vi "test_F9P.vi"() -> ()   [LabVIEW 2019] (continued)
085,36,09,44,196,30,11,78,037,33,2*7B\r\n$GAGSV,3,2,09,12,32,115,24,18,55,284,37,19,17,042,30,25,01,241,,2*76\r\n$GAGSV,3,3,09,36,35,314,26,2*4E\r\n$GBGSV,4,1,13,04,35,133,,05,09,257,,06,27,182,,07,09,201,,1*7B\r\n$GBGSV,4,2,13,08,65,355,39,09,07,194,,10,16,222,23,11,37,142,25,1*73\r\n$GBGSV,4,3,13,13,50,315,40,14,76,037,42,28,59,310,38,33,73,239,30,1*71\r\n$GBGSV,4,4,13,34,13,142,,1*46\r\n$GBGSV,4,1,13,04,35,133,,05,09,257,,06,27,182,,07,09,201,,3*79\r\n$GBGSV,4,2,13,08,65,355,38,09,07,194,,10,16,222,26,11,37,142,35,3*74\r\n$GBGSV,4,3,13,13,50,315,42,14,76,037,38,28,59,310,,33,73,239,,3*74\r\n$GBGSV,4,4,13,34,13,142,,3*44\r\n$GNGLL,3723.61677,N,12656.96875,E,064301.00,A,A*70\r\n$GNRMC,064302.00,A,3723.61678,N,12656.96879,E,0.043,,250720,,,A,V*16\r\n$GNVTG,,T,,M,0.043,N,0.079,K,A*34\r\n$GNGGA,064302.00,3723.61678,N,12656.96879,E,1,12,0.63,44.0,M,18.5,M,,*7F\r\n$GNGSA,A,3,17,19,06,05,02,12,09,,,,,,1.10,0.63,0.91,1*09\r\n$GNGSA,A,3,85,70,71,72,,,,,,,,,1.10,0.63,0.91,2*06\r\n$GNGSA,A,3,36,19,11,04,09,12,,,,,,,1.10,0.63,0.91,3*0D\r\n$GNGSA,A,3,28,14,13,11,33,08,10,,,,,,1.10,0.63,0.91,4*0D\r\n$GPGSV,4,1,13,02,65,334,45,04,08,037,36,05,48,261,35,06,58,076,45,1*6B\r\n$GPGSV,4,2,13,07,06,105,,09,38,057,49,12,18,263,22,13,08,191,21,1*65\r\n$GPGSV,4,3,13,17,19,158,26,19,37,161,28,25,11,294,,29,07,323,21,1*62\r\n$GPGSV,4,4,13,30,01,134,,1*52\r\n$GPGSV,4,1,13,02,65,334,,04,08,037,21,05,48,261,32,06,58,076,24,6*6B\r\n$GPGSV,4,2,13,07,06,105,10,09,38,057,40,12,18,263,12,13,08,191,,6*6A\r\n$GPGSV,4,3,13,17,19,158,17,19,37,161,,25,11,294,,29,07,323,,6*6E\r\n$GPGSV,4,4,13,30,01,134,,6*55\r\n$GLGSV,2,1,06,70,55,030,38,71,68,223,32,72,17,216,36,84,09,133,12,1*7C\r\n$GLGSV,2,2,06,85,63,111,36,86,51,337,,1*7F\r\n$GLGSV,2,1,06,70,55,030,,71,68,223,18,72,17,216,22,84,09,133,12,3*78\r\n$GLGSV,2,2,06,85,63,111,28,86,51,337,19,3*7A\r\n$GAGSV,3,1,09,02,04,287,09,04,68,085,42,09,44,196,31,11,78,037,39,7*7F\r\n$GAGSV,3,2,09,12,32,115,28,18,55,284,35,19,17,042,34,25,01,241,,7*79\r\n$GAGSV,3,3,09,36,35,314,33,7*4F\r\n$GAGSV,3,1,09,02,04,287,,04,68,085,36,09,44,196,26,11,78,037,33,2*7C\r\n$GAGSV,3,2,09,12,32,115,24,18,55,284,38,19,17,042,30,25,01,241,,2*79\r\n$GAGSV,3,3,09,36,35,314,26,2*4E\r\n$GBGSV,4,1,13,04,35,133,,05,09,257,,06,27,182,,07,09,201,,1*7B\r\n$GBGSV,4,2,13,08,65,355,40,09,07,194,,10,16,222,22,11,37,142,22,1*7B\r\n$GBGSV,4,3,13,13,50,315,40,14,76,037,42,28,59,310,38,33,73,239,32,1*73\r\n$GBGSV,4,4,13,34,13,142,,1*46\r\n$GBGSV,4,1,13,04,35,133,,05,09,257,,06,27,182,,07,09,201,,3*79\r\n$GBGSV,4,2,13,08,65,355,38,09,07,194,,10,16,222,26,11,37,142,34,3*75\r\n$GBGSV,4,3,13,13,50,315,41,14,76,037,37,28,59,310,,33,73,239,,3*78\r\n$GBGSV,4,4,13,34,13,142,,3*44\r\n$GNGLL,3723.61678,N,12656.96879,E,064302.00,A,A*70\r\n$GNRMC,064303.00,A,3723.61679,N,12656.96883,E,0.052,,250720,,,A,V*13\r\n$GNVTG,,T,,M,0.052,N,0.096,K,A*35\r\n$GNGGA,064303.00,3723.61679,N,12656.96883,E,1,12,0.63,44.1,M,18.5,M,,*7B\r\n$GNGSA,A,3,17,19,06,05,02,12,09,,,,,,1.10,0.63,0.91,1*09\r\n$GNGSA,A,3,85,70,71,72,,,,,,,,,1.10,0.63,0.91,2*06\r\n$GNGSA,A,3,36,19,11,04,09,12,,,,,,,1.10,0.63,0.91,3*0D\r\n$GNGSA,A,3,28,14,13,11,33,08,10,,,,,,1.10,0.63,0.91,4*0D\r\n$GPGSV,4,1,13,02,65,334,44,04,08,037,33,05,48,261,31,06,58,076,44,1*6A\r\n$GPGSV,4,2,13,07,06,105,,09,38,057,49,12,18,263,22,13,08,191,21,1*65\r\n$GPGSV,4,3,13,17,19,158,26,19,37,161,28,25,11,294,,29,07,323,20,1*63\r\n$GPGSV,4,4,13,30,01,134,,1*52\r\n$GPGSV,4,1,13,02,65,334,,04,08,037,22,05,48,261,32,06,58,076,26,6*6A\r\n$GPGSV,4,2,13,07,06,105,08,09,38,057,40,12,18,263,12,13,08,191,,6*63\r\n$GPGSV,4,3,13,17,19,158,17,19,37,161,,25,11,294,,29,07,323,,6*6E\r\n$GPGSV,4,4,13,30,01,134,,6*55\r\n$GLGSV,2,1,06,70,55,030,36,71,68,223,35,72,17,216,36,84,09,133,09,1*7F\r\n$GLGSV,2,2,06,85,63,111,37,86,51,337,,1*7E\r\n$GLGSV,2,1,06,70,55,030,,71,68,223,16,72,17,216,21,84,09,133,13,3*74\r\n$GLGSV,2,2,06,85,63,111,29,86,51,337,17,3*75\r\n$GAGSV,3,1,09,02,04,287,07,04,68,085,42,09,44,196,31,11,78,037,39,7*71\r\n$GAGSV,3,2,09,12,32,115,30,18,55,284,37,19,17,042,37,25,01,241,,7*71\r\n$GAGSV,3,3,09,36,35,314,34,7*48\r\n$GAGSV,3,1,09,02,04,287,,04,68,085,36,09,44,196,27,11,78,037,33,2*7D\r\n$GAGSV,3,2,09,12,32,115,24,18,55,284,38,19,17,042,31,25,01,241,,2*78\r\n$GAGSV,3,3,09,36,35,314,26,2*4E\r\n$GBGSV,4,1,13,04,35,133,,05,09,257,,06,27,182,,07,09,201,,1*7B\r\n$GBGSV,4,2,13,08,65,355,39,09,07,194,,10,16,222,21,11,37,142,22,1*76\r\n$GBGSV,4,3,13,13,50,315,40,14,76,037,43,28,59,310,38,33,73,239,28,1*79\r\n$GBGSV,4,4,13,34,13,142,,1*46\r\n$GBGSV,4,1,13,04,35,133,,05,09,257,,06,27,182,,07,09,201,,3*79\r\n$GBGSV,4,2,13,08,65,355,36,09,07,194,,10,16,222,25,11,37,142,34,3*78\r\n$GBGSV,4,3,13,13,50,315,40,14,76,037,37,28,59,310,,33,73,239,,3*79\r\n$GBGSV,4,4,13,34,13,142,,3*44\r\n$GNGLL,3723.61679,N,12656.96883,E,064303.00,A,A*75\r\n$GNRMC,064304.00,A,3723.61678,N,12656.96886,E,0.034,,250720,,,A,V*10\r\n$GNVTG,,T,,M,0.034,N,0.063,K,A*3F\r\n$GNGGA,064304.00,3723.61678,N,12656.96886,E,1,12,0.66,44.1,M,18.5,M,,*7D\r\n$GNGSA,A,3,17,19,06,05,02,12,09,,,,,,1.18,0.66,0.98,1*0D\r\n$GNGSA,A,3,85,70,71,72,,,,,,,,,1.18,0.66,0.98,2*02\r\n$GNGSA,A,3,36,19,11,04,09,12,,,,,,,1.18,0.66,0.98,3*09\r\n$GNGSA,A,3,28,14,13,11,33,08,10,,,,,,1.18,0.66,0.98,4*09\r\n$GPGSV,4,1,13,02,65,334,45,04,08,037,28,05,48,261,34,06,58,076,43,1*63\r\n$GPGSV,4,2,13,07,06,105,26,09,38,057,47,12,18,263,24,13,08,191,20,1*68\r\n$GPGSV,4,3,13,17,19,158,26,19,37,161,26,25,11,294,,29,07,323,19,1*67\r\n$GPGSV,4,4,13,30,01,134,,1*52\r\n$GPGSV,4,1,13,02,65,334,,04,08,037,25,05,48,261,32,06,58,076,28,6*63\r\n$GPGSV,4,2,13,07,06,105,,09,38,057,40,12,18,263,14,13,08,191,,6*6D\r\n$GPGSV,4,3,13,17,19,158,17,19,37,161,,25,11,294,,29,07,323,,6*6E\r\n$GPGSV,4,4,13,30,01,134,,6*55\r\n$GLGSV,2,1,06,70,54,030,35,71,68,223,36,72,17,216,36,84,09,133,08,1*7F\r\n$GLGSV,2,2,06,85,63,111,39,86,51,337,,1*70\r\n$GLGSV,2,1,06,70,54,030,,71,68,223,14,72,17,216,21,84,09,133,10,3*74\r\n$GLGSV,2,2,06,85,63,111,28,86,51,337,15,3*76\r\n$GAGSV,3,1,09,02,04,287,10,04,68,085,42,09,44,196,31,11,78,037,39,7*77\r\n$GAGSV,3,2,09,12,32,115,30,18,55,284,34,19,17,042,36,25,01,241,,7*73\r\n$GAGSV,3,3,09,36,35,314,33,7*4F\r\n$GAGSV,3,1,09,02,04,287,,04,68,085,35,09,44,196,28,11,78,037,33,2*71\r\n$GAGSV,3,2,09,12,32,115,24,18,55,284,38,19,17,042,31,25,01,241,,2*78\r\n$GAGSV,3,3,09,36,35,314,26,2*4E\r\n$GBGSV,4,1,13,04,35,133,,05,09,257,,06,27,182,,07,09,201,,1*7B\r\n$GBGSV,4,2,13,08,65,355,40,09,07,194,,10,16,222,21,11,37,142,21,1*7B\r\n$GBGSV,4,3,13,13,50,315,39,14,76,037,43,28,59,310,38,33,73,239,28,1*77\r\n$GBGSV,4,4,13,34,13,142,,1*46\r\n$GBGSV,4,1,13,04,35,133,,05,09,257,,06,27,182,,07,09,201,,3*79\r\n$GBGSV,4,2,13,08,65,355,36,09,07,194,,10,16,222,25,11,37,142,33,3*7F\r\n$GBGSV,4,3,13,13,50,315,41,14,76,037,37,28,59,310,,33,73,239,,3*78\r\n$GBGSV,4,4,13,34,13,142,,3*44\r\n$GNGLL,3723.61678,N,12656.96886,E,064304.00,A,A*76\r\n$GNRMC,064305.00,A,3723.61669,N,12656.96881,E,0.430,127.96,250720,,,A,V*03\r\n$GNVTG,127.96,T,,M,0.430,N,0.797,K,A*26\r\n$GNGGA,064305.00,3723.61669,N,12656.96881,E,1,12,0.66,43.9,M,18.5,M,,*74\r\n$GNGSA,A,3,17,19,06,05,02,12,09,,,,,,1.18,0.66,0.98,1*0D\r\n$GNGSA,A,3,85,70,71,72,,,,,,,,,1.18,0.66,0.98,2*02\r\n$GNGSA,A,3,36,19,11,04,09,12,,,,,,,1.18,0.66,0.98,3*09\r\n$GNGSA,A,3,28,14,13,11,33,08,10,,,,,,1.18,0.66,0.98,4*09\r\n$GPGSV,4,1,13,02,65,334,46,04,08,037,26,05,48,261,39,06,58,076,45,1*65\r\n$GPGSV,4,2,13,07,06,105,,09,38,057,47,12,18,263,22,13,08,191,18,1*61\r\n$GPGSV,4,3,13,17,19,158,25,19,37,161,24,25,11,294,,29,07,323,17,1*68\r\n$GPGSV,4,4,13,30,01,134,,1*52\r\n$GPGSV,4,1,13,02,65,334,,04,08,037,29,05,48,261,33,06,58,076,30,6*67\r\n$GPGSV,4,2,13,07,06,105,,09,38,057,40,12,18,263,13,13,08,191,,6*6A\r\n$GPGSV,4,3,13,17,19,158,16,19,37,161,,25,11,294,,29,07,323,,6*6F\r\n$GPGSV,4,4,13,30,01,134,,6*55\r\n$GLGSV,2,1,06,70,54,030,32,71,69,224,36,72,17,216,38,84,09,133,10,1*79\r\n$GLGSV,2,2,06,85,63,111,40,86,51,337,,1*7E\r\n$GLGSV,2,1,06,70,54,030,,71,69,224,11,72,17,216,23,84,09,133,10,3*75\r\n$GLGSV,2,2,06,85,63,111,29,86,51,337,12,3*70\r\n$GAGSV,3,1,09,02,04,287,08,04,68,085,43,09,44,196,29,11,78,037,39,7*76\r\n$GAGSV,3,2,09,12,32,115,30,18,55,284,30,19,17,042,33,25,01,241,,7*72\r\n$GAGSV,3,3,09,36,35,314,33,7*4F\r\n$GAGSV,3,1,09,02,04,287,,04,68,085,38,09,44,196,27,11,78,037,34,2*74\r\n$GAGSV,3,2,09,12,32,115,26,18,55,284,37,19,17,042,26,25,01,241,,2*73\r\n$GAGSV,3,3,09,36,35,314,26,2*4E\r\n$GBGSV,4,1,13,04,35,133,,05,09,257,,06,27,182,,07,09,201,,1*7B\r\n$GBGSV,4,2,13,08,65,355,40,09,07,194,,10,16,222,20,11,37,142,21,1*7A\r\n$GBGSV,4,3,13,13,50,315,39,14,76,037,42,28,59,310,38,33,73,239,31,1*7E\r\n$GBGSV,4,4,13,34,13,142,,1*46\r\n$GBGSV,4,1,13,04,35,133,,05,09,257,,06,27,182,,07,09,201,,3*79\r\n$GBGSV,4,2,13,08,65,355,36,09,07,194,,10,16,222,25,11,37,142,33,3*7F\r\n$GBGSV,4,3,13,13,50,315,41,14,76,037,38,28,59,310,,33,73,239,,3*77\r\n$GBGSV,4,4,13,34,13,142,,3*44\r\n$GNGLL,3723.61669,N,12656.96881,E,064305.00,A,A*70\r\n$GNRMC,064306.00,A,3723.61673,N,12656.96884,E,0.012,,250720,,,A,V*1F\r\n$GNVTG,,T,,M,0.012,N,0.023,K,A*3F\r\n$GNGGA,064306.00,3723.61673,N,12656.96884,E,1,12,0.62,44.0,M,18.5,M,,*73\r\n$GNGSA,A,3,17,19,06,05,02,12,09,,,,,,1.09,0.62,0.90,1*01\r\n$GNGSA,A,3,85,70,71,72,,,,,,,,,1.09,0.62,0.90,2*0E\r\n$GNGSA,A,3,36,19,11,04,09,12,,,,,,,1.09,0.62,0.90,3*05\r\n$GNGSA,A,3,28,14,13,11,33,08,10,,,,,,1.09,0.62,0.90,4*05\r\n$GPGSV,4,1,13,02,65,334,45,04,08,037,33,05,48,261,33,06,58,076,43,1*6E\r\n$GPGSV,4,2,13,07,06,105,,09,38,057,47,12,18,263,25,13,08,191,16,1*68\r\n$GPGSV,4,3,13,17,19,158,26,19,37,161,23,25,11,294,,29,07,323,17,1*6C\r\n$GPGSV,4,4,13,30,01,134,,1*52\r\n$GPGSV,4,1,13,02,65,334,,04,08,037,24,05,48,261,34,06,58,076,29,6*65\r\n$GPGSV,4,2,13,07,06,105,,09,38,057,40,12,18,263,10,13,08,191,,6*69\r\n$GPGSV,4,3,13,17,19,158,19,19,37,161,,25,11,294,,29,07,323,,6*60\r\n$GPGSV,4,4,13,30,01,134,,6*55\r\n$GLGSV,2,1,06,70,54,030,37,71,69,224,36,72,18,217,36,84,09,133,11,1*7D\r\n$GLGSV,2,2,06,85,63,111,40,86,51,337,,1*7E\r\n$GLGSV,2,1,06,70,54,030,,71,69,224,08,72,18,217,24,84,09,133,09,3*7C\r\n$GLGSV,2,2,06,85,63,111,30,86,51,337,09,3*72\r\n$GAGSV,3,1,09,02,04,287,10,04,68,085,43,09,44,196,32,11,78,037,39,7*75\r\n$GAGSV,3,2,09,12,32,115,29,18,55,284,37,19,17,042,33,25,01,241,,7*7D\r\n$GAGSV,3,3,09,36,35,314,33,7*4F\r\n$GAGSV,3,1,09,02,04,287,,04,68,085,36,09,44,196,27,11,78,037,33,2*7D\r\n$GAGSV,3,2,09,12,32,115,24,18,55,284,37,19,17,042,31,25,01,241,,2*77\r\n$GAGSV,3,3,09,36,35,314,25,2*4D\r\n$GBGSV,4,1,13,04,35,133,,05,09,257,,06,27,182,,07,09,201,,1*7B\r\n$GBGSV,4,2,13,08,65,355,40,09,07,194,,10,16,222,19,11,37,142,20,1*71\r\n$GBGSV,4,3,13,13,50,315,39,14,76,037,43,28,59,310,38,33,73,239,31,1*7F\r\n$GBGSV,4,4,13,34,13,142,,1*46\r\n$GBGSV,4,1,13,04,35,133,,05,09,257,,06,27,182,,07,09,201,,3*79\r\n$GBGSV,4,2,13,08,65,355,36,09,07,194,,10,16,222,25,11,37,142,34,3*78\r\n$GBGSV,4,3,13,13,50,315,40,14,76,037,36,28,59,310,,33,73,239,,3*78\r\n$GBGSV,4,4,13,34,13,142,,3*44\r\n$GNGLL,3723.61673,N,12656.96884,E,064306.00,A,A*7D\r\n$GNRMC,064307.00,A,3723.61674,N,12656.96886,E,0.029,,250720,,,A,V*13\r\n$GNVTG,,T,,M,0.029,N,0.053,K,A*30\r\n$GNGGA,064307.00,3723.61674,N,12656.96886,E,1,12,0.62,44.0,M,18.5,M,,*77\r\n$GNGSA,A,3,17,19,06,05,02,12,09,,,,,,1.09,0.62,0.90,1*01\r\n$GNGSA,A,3,85,70,71,72,,,,,,,,,1.09,0.62,0.90,2*0E\r\n$GNGSA,A,3,36,19,11,04,09,12,,,,,,,1.09,0.62,0.90,3*05\r\n$GNGSA,A,3,28,14,13,11,33,08,10,,,,,,1.09,0.62,0.90,4*05\r\n$GPGSV,4,1,13,02,65,334,46,04,08,037,37,05,48,261,33,06,58,076,44,1*6E\r\n$GPGSV,4,2,13,07,06,105,,09,38,057,48,12,18,263,25,13,08,191,,1*60\r\n$GPGSV,4,3,13,17,19,158,26,19,37,161,24,25,11,294,,29,07,323,21,1*6E\r\n$GPGSV,4,4,13,30,01,134,,1*52\r\n$GPGSV,4,1,13,02,65,334,,04,08,037,23,05,48,261,33,06,58,076,28,6*64\r\n$GPGSV,4,2,13,07,06,105,,09,38,057,41,12,18,263,,13,08,191,,6*69\r\n$GPGSV,4,3,13,17,19,158,19,19,37,161,,25,11,294,,29,07,323,,6*60\r\n$GPGSV,4,4,13,30,01,134,,6*55\r\n$GLGSV,2,1,06,70,54,030,36,71,69,224,36,72,18,217,35,84,09,133,11,1*7F\r\n$GLGSV,2,2,06,85,63,111,39,86,51,337,,1*70\r\n$GLGSV,2,1,06,70,54,030,,71,69,224,07,72,18,217,24,84,09,133,10,3*7B\r\n$GLGSV,2,2,06,85,63,111,29,86,51,337,09,3*7A\r\n$GAGSV,3,1,09,02,04,287,11,04,68,085,43,09,44,196,31,11,78,037,40,7*79\r\n$GAGSV,3,2,09,12,32,115,28,18,55,284,37,19,17,042,33,25,01,241,,7*7C\r\n$GAGSV,3,3,09,36,35,314,34,7*48\r\n$GAGSV,3,1,09,02,04,287,,04,68,085,36,09,44,196,28,11,78,037,33,2*72\r\n$GAGSV,3,2,09,12,32,115,25,18,55,284,38,19,17,042,30,25,01,241,,2*78\r\n$GAGSV,3,3,09,36,35,314,25,2*4D\r\n$GBGSV,4,1,13,04,35,133,,05,09,257,,06,27,182,,07,09,201,,1*7B\r\n$GBGSV,4,2,13,08,65,355,40,09,07,194,,10,16,222,20,11,37,142,21,1*7A\r\n$GBGSV,4,3,13,13,50,315,40,14,76,037,42,28,59,310,39,33,73,239,30,1*70\r\n$GBGSV,4,4,13,34,13,142,20,1*44\r\n$GBGSV,4,1,13,04,35,133,,05,09,257,,06,27,182,,07,09,201,,3*79\r\n$GBGSV,4,2,13,08,65,355,37,09,07,194,,10,16,222,25,11,37,142,34,3*79\r\n$GBGSV,4,3,13,13,50,315,40,14,76,037,36,28,59,310,,33,73,239,,3*78\r\n$GBGSV,4,4,13,34,13,142,,3*44\r\n$GNGLL,3723.61674,N,12656.96886,E,064307.00,A,A*79\r\n$GNRMC,064308.00,A,3723.61673,N,12656.96888,E,0.031,,250720,,,A,V*1C\r\n$GNVTG,,T,,M,0.031,N,0.057,K,A*3D\r\n$GNGGA,064308.00,3723.61673,N,12656.96888,E,1,12,0.62,44.0,M,18.5,M,,*71\r\n$GNGSA,A,3,17,19,06,05,02,12,09,,,,,,1.09,0.62,0.90,1*01\r\n$GNGSA,A,3,85,70,71,72,,,,,,,,,1.09,0.62,0.90,2*0E\r\n$GNGSA,A,3,36,19,11,04,09,12,,,,,,,1.09,0.62,0.90,3*05\r\n$GNGSA,A,3,28,14,13,11,33,08,10,,,,,,1.09,0.62,0.90,4*05\r\n$GPGSV,4,1,13,02,65,334,46,04,08,037,34,05,48,261,34,06,58,076,45,1*6B\r\n$GPGSV,4,2,13,07,06,105,,09,38,057,47,12,18,263,26,13,08,191,20,1*6E\r\n$GPGSV,4,3,13,17,19,158,26,19,37,161,24,25,11,294,,29,07,323,22,1*6D\r\n$GPGSV,4,4,13,30,01,134,,1*52\r\n$GPGSV,4,1,13,02,65,334,,04,08,037,25,05,48,261,33,06,58,076,29,6*63\r\n$GPGSV,4,2,13,07,06,105,,09,38,057,39,12,18,263,,13,08,191,,6*66\r\n$GPGSV,4,3,13,17,19,158,19,19,37,161,,25,11,294,,29,07,323,,6*60\r\n$GPGSV,4,4,13,30,01,134,,6*55\r\n$GLGSV,2,1,06,70,54,030,36,71,69,224,36,72,18,217,37,84,09,133,13,1*7F\r\n$GLGSV,2,2,06,85,63,111,40,86,51,337,,1*7E\r\n$GLGSV,2,1,06,70,54,030,,71,69,224,13,72,18,217,23,84,09,133,16,3*7F\r\n$GLGSV,2,2,06,85,63,111,30,86,51,337,11,3*7B\r\n$GAGSV,3,1,09,02,04,287,10,04,68,085,43,09,44,196,31,11,78,037,40,7*78\r\n$GAGSV,3,2,09,12,32,115,27,18,55,284,36,19,17,042,29,25,01,241,,7*79\r\n$GAGSV,3,3,09,36,35,314,33,7*4F\r\n$GAGSV,3,1,09,02,04,287,,04,68,085,36,09,44,196,28,11,78,037,32,2*73\r\n$GAGSV,3,2,09,12,32,115,24,18,55,284,38,19,17,042,,25,01,241,,2*7A\r\n$GAGSV,3,3,09,36,35,314,24,2*4C\r\n$GBGSV,4,1,13,04,35,133,,05,09,257,,06,27,182,,07,09,201,,1*7B\r\n$GBGSV,4,2,13,08,65,355,40,09,07,194,,10,16,222,20,11,37,142,23,1*78\r\n$GBGSV,4,3,13,13,50,315,40,14,76,037,42,28,59,310,38,33,73,239,30,1*71\r\n$GBGSV,4,4,13,34,13,142,21,1*45\r\n$GBGSV,4,1,13,04,35,133,,05,09,257,,06,27,182,,07,09,201,,3*79\r\n$GBGSV,4,2,13,08,65,355,37,09,07,194,,10,16,222,25,11,37,142,34,3*79\r\n$GBGSV,4,3,13,13,50,315,41,14,76,037,37,28,59,310,,33,73,239,,3*78\r\n$GBGSV,4,4,13,34,13,142,,3*44\r\n$GNGLL,3723.61673,N,12656.96888,E,064308.00,A,A*7F\r\n$GNRMC,064309.00,A,3723.61674,N,12656.96889,E,0.064,,250720,,,A,V*1B\r\n$GNVTG,,T,,M,0.064,N,0.119,K,A*36\r\n$GNGGA,064309.00,3723.61674,N,12656.96889,E,1,12,0.62,44.1,M,18.5,M,,*77\r\n$GNGSA,A,3,17,19,06,05,02,12,09,,,,,,1.09,0.62,0.90,1*01\r\n$GNGSA,A,3,85,70,71,72,,,,,,,,,1.09,0.62,0.90,2*0E\r\n$GNGSA,A,3,36,19,11,04,09,12,,,,,,,1.09,0.62,0.90,3*05\r\n$GNGSA,A,3,28,14,13,11,33,08,34,10,,,,,1.09,0.62,0.90,4*02\r\n$GPGSV,4,1,13,02,65,334,46,04,08,037,38,05,48,261,34,06,58,076,44,1*66\r\n$GPGSV,4,2,13,07,06,105,,09,38,057,47,12,18,263,25,13,08,191,20,1*6D\r\n$GPGSV,4,3,13,17,19,158,28,19,37,161,24,25,11,294,,29,07,323,23,1*62\r\n$GPGSV,4,4,13,30,01,134,,1*52\r\n$GPGSV,4,1,13,02,65,334,,04,08,037,25,05,48,261,33,06,58,076,28,6*62\r\n$GPGSV,4,2,13,07,06,105,,09,38,057,41,12,18,263,,13,08,191,,6*69\r\n$GPGSV,4,3,13,17,19,158,19,19,37,161,,25,11,294,,29,07,323,,6*60\r\n$GPGSV,4,4,13,30,01,134,,6*55\r\n$GLGSV,2,1,06,70,54,030,36,71,69,224,36,72,18,217,35,84,09,133,18,1*76\r\n$GLGSV,2,2,06,85,63,111,41,86,51,337,,1*7F\r\n$GLGSV,2,1,06,70,54,030,,71,69,224,15,72,18,217,24,84,09,133,15,3*7D\r\n$GLGSV,2,2,06,85,63,111,30,86,51,337,,3*7B\r\n$GAGSV,3,1,09,02,04,287,07,04,68,085,44,09,44,196,31,11,78,037,40,7*79\r\n$GAGSV,3,2,09,12,32,115,26,18,55,284,36,19,17,042,34,25,01,241,,7*74\r\n$GAGSV,3,3,09,36,35,314,33,7*4F\r\n$GAGSV,3,1,09,02,04,287,,04,68,085,36,09,44,196,29,11,78,037,33,2*73\r\n$GAGSV,3,2,09,12,32,115,25,18,55,284,38,19,17,042,29,25,01,241,,2*70\r\n$GAGSV,3,3,09,36,35,314,24,2*4C\r\n$GBGSV,4,1,13,04,35,133,,05,09,257,,06,27,182,,07,09,201,,1*7B\r\n$GBGSV,4,2,13,08,65,355,40,09,07,194,,10,16,222,19,11,37,142,24,1*75\r\n$GBGSV,4,3,13,13,50,315,40,14,76,037,42,28,59,310,39,33,73,239,31,1*71\r\n$GBGSV,4,4,13,34,13,142,22,1*46\r\n$GBGSV,4,1,13,04,35,133,,05,09,257,,06,27,182,,07,09,201,,3*79\r\n$GBGSV,4,2,13,08,65,355,37,09,07,194,,10,16,222,24,11,37,142,35,3*79\r\n$GBGSV,4,3,13,13,50,315,41,14,76,037,37,28,59,310,,33,73,239,,3*78\r\n$GBGSV,4,4,13,34,13,142,,3*44\r\n$GNGLL,3723.61674,N,12656.96889,E,064309.00,A,A*78\r\n$GNRMC,064310.00,A,3723.61678,N,12656.96893,E,0.073,,250720,,,A,V*12\r\n$GNVTG,,T,,M,0.073,N,0.136,K,A*3D\r\n$GNGGA,064310.00,3723.61678,N,12656.96893,E,1,12,0.62,44.1,M,18.5,M,,*78\r\n$GNGSA,A,3,17,19,06,05,02,12,09,,,,,,1.09,0.62,0.90,1*01\r\n$GNGSA,A,3,85,70,71,72,,,,,,,,,1.09,0.62,0.90,2*0E\r\n$GNGSA,A,3,36,19,11,04,09,12,,,,,,,1.09,0.62,0.90,3*05\r\n$GNGSA,A,3,28,14,13,11,33,08,10,,,,,,1.09,0.62,0.90,4*05\r\n$GPGSV,4,1,13,02,65,334,46,04,08,037,39,05,48,261,32,06,58,076,44,1*61\r\n$GPGSV,4,2,13,07,06,105,,09,38,057,44,12,18,263,25,13,08,191,19,1*64\r\n$GPGSV,4,3,13,17,19,158,28,19,37,161,24,25,11,294,,29,07,323,22,1*63\r\n$GPGSV,4,4,13,30,01,134,,1*52\r\n$GPGSV,4,1,13,02,65,334,,04,08,037,24,05,48,261,36,06,58,076,30,6*6F\r\n$GPGSV,4,2,13,07,06,105,,09,38,057,39,12,18,263,,13,08,191,,6*66\r\n$GPGSV,4,3,13,17,19,158,20,19,37,161,,25,11,294,,29,07,323,,6*6A\r\n$GPGSV,4,4,13,30,01,134,,6*55\r\n$GLGSV,2,1,06,70,54,030,36,71,69,224,35,72,18,217,38,84,09,133,14,1*74\r\n$GLGSV,2,2,06,85,63,111,39,86,51,337,,1*70\r\n$GLGSV,2,1,06,70,54,030,,71,69,224,13,72,18,217,26,84,09,133,17,3*7B\r\n$GLGSV,2,2,06,85,63,111,30,86,51,337,,3*7B\r\n$GAGSV,3,1,09,02,04,287,10,04,68,085,44,09,44,196,30,11,78,037,40,7*7E\r\n$GAGSV,3,2,09,12,32,115,25,18,55,284,36,19,17,042,33,25,01,241,,7*70\r\n$GAGSV,3,3,09,36,35,314,33,7*4F\r\n$GAGSV,3,1,09,02,04,287,,04,68,085,36,09,44,196,29,11,78,037,32,2*72\r\n$GAGSV,3,2,09,12,32,115,26,18,55,284,38,19,17,042,32,25,01,241,,2*79\r\n$GAGSV,3,3,09,36,35,314,24,2*4C\r\n$GBGSV,4,1,13,04,35,133,,05,09,257,,06,27,182,,07,09,201,,1*7B\r\n$GBGSV,4,2,13,08,65,355,40,09,07,194,,10,16,222,19,11,37,142,23,1*72\r\n$GBGSV,4,3,13,13,50,315,40,14,76,037,42,28,59,310,39,33,73,239,30,1*70\r\n$GBGSV,4,4,13,34,13,142,,1*46\r\n$GBGSV,4,1,13,04,35,133,,05,09,257,,06,27,182,,07,09,201,,3*79\r\n$GBGSV,4,2,13,08,65,355,37,09,07,194,,10,16,222,24,11,37,142,34,3*78\r\n$GBGSV,4,3,13,13,50,315,41,14,76,037,36,28,59,310,,33,73,239,,3*79\r\n$GBGSV,4,4,13,34,13,142,,3*44\r\n$GNGLL,3723.61678,N,12656.96893,E,064310.00,A,A*77\r\n$GNRMC,064311.00,A,3723.61684,N,12656.96898,E,0.051,,250720,,,A,V*1B\r\n$GNVTG,,T,,M,0.051,N,0.095,K,A*35\r\n$GNGGA,064311.00,3723.61684,N,12656.96898,E,1,12,0.62,44.3,M,18.5,M,,*73\r\n$GNGSA,A,3,17,19,06,05,02,12,09,,,,,,1.09,0.62,0.90,1*01\r\n$GNGSA,A,3,85,70,71,72,,,,,,,,,1.09,0.62,0.90,2*0E\r\n$GNGSA,A,3,36,19,11,04,09,12,,,,,,,1.09,0.62,0.90,3*05\r\n$GNGSA,A,3,28,14,13,11,33,08,10,,,,,,1.09,0.62,0.90,4*05\r\n$GPGSV,4,1,13,02,65,334,46,04,08,037,37,05,48,261,36,06,58,076,45,1*6A\r\n$GPGSV,4,2,13,07,06,105,,09,38,057,46,12,18,263,26,13,08,191,19,1*65\r\n$GPGSV,4,3,13,17,19,158,29,19,37,161,23,25,11,294,,29,07,323,22,1*65\r\n$GPGSV,4,4,13,30,01,134,,1*52\r\n$GPGSV,4,1,13,02,65,334,,04,08,037,24,05,48,261,33,06,58,076,30,6*6A\r\n$GPGSV,4,2,13,07,06,105,,09,38,057,40,12,18,263,,13,08,191,,6*68\r\n$GPGSV,4,3,13,17,19,158,19,19,37,161,,
